vi "HandleRanges.vi"(0 "reference in":refnum<class "Sig_AI.lvclass">, 11 "error in (no error)":errorcluster) -> (4 "reference out":refnum<class "Sig_AI.lvclass">, 15 "error out":errorcluster)   [LabVIEW 2019, in "Sig_AI.lvclass"]
uses:
  Sig_AI.lvclass
  Sig_AI.lvclass/Sig_AI.ctl
  AnalogComparator_class/AnalogComparator.lvclass/AnalogComparator.ctl
  AnalogComparator_class/HandleDb.vi
  AnalogComparator_class/AnalogComparator.lvclass
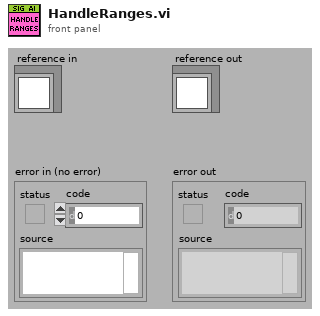
[diagram p1: front panel]
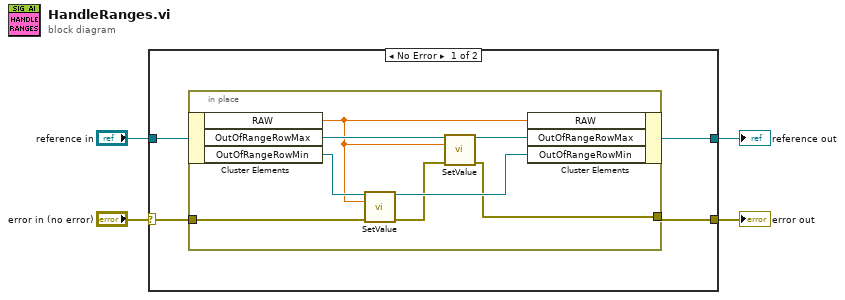
[diagram p0: block diagram]
diagram:
  n1 = case shown="No Error" "error in (no error)" {
    selector: "error in (no error)" -> [w6 w18]
    tunnel: [w5 w18] -> w3
    tunnel: [w7 w17] -> w1
    tunnel: "reference in" -> [w8 w17]
    frame No Error {
      n2 = in-place {
        in-place-border: w6 -> [w11]
        in-place-border: [w9] -> w5
        n3 = in-place-cluster #1(w8) -> ("RAW"=w13:dbl, "OutOfRangeRowMax"=w16:refnum<class "AnalogComparator.lvclass">, "OutOfRangeRowMin"=w14:refnum<class "AnalogComparator.lvclass">)
        n4 = call "SetValue.vi"("class data in"=w14, "Value"=w13, "error in (no error)"=w11) -> ("class data out"=w12:refnum<class "AnalogComparator.lvclass">, "error out"=w10:errorcluster)  [unwired: 11 in]
        n5 = call "SetValue.vi"("class data in"=w16, "Value"=w13, "error in (no error)"=w10) -> ("class data out"=w15:refnum<class "AnalogComparator.lvclass">, "error out"=w9:errorcluster)  [unwired: 11 in]
        n6 = in-place-cluster #1("RAW"=w13, "OutOfRangeRowMax"=w15, "OutOfRangeRowMin"=w12) -> (w7:refnum<class "Sig_AI.lvclass">)
      }
    }
    frame Error {
    }
  }
  "error out" <- w3
  "reference out" <- w1
